vi "Create 2D Gauss.vi"(4 "Rauschen %":dbl=10.0, 6 "1/e HWidth":dbl, 7 "Y size":i32, 8 "mitte y":dbl, 9 "mitte x":dbl, 10 "Order":dbl, 11 "X size":i32) -> (1 "Total Count":sgl, 3 "2D Gauss":sgl[][](array[numeric]))   [LabVIEW 2020, in "Camera Simulator.lvlib"]
uses:
  Camera Simulator.lvlib
  <vilib>/numeric/Random Number (Range) DBL.vi
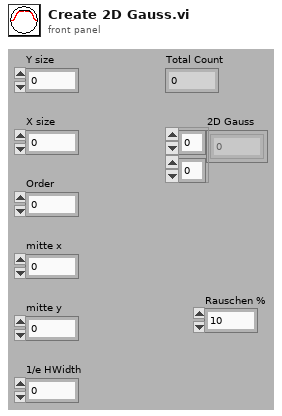
[diagram p1: front panel]
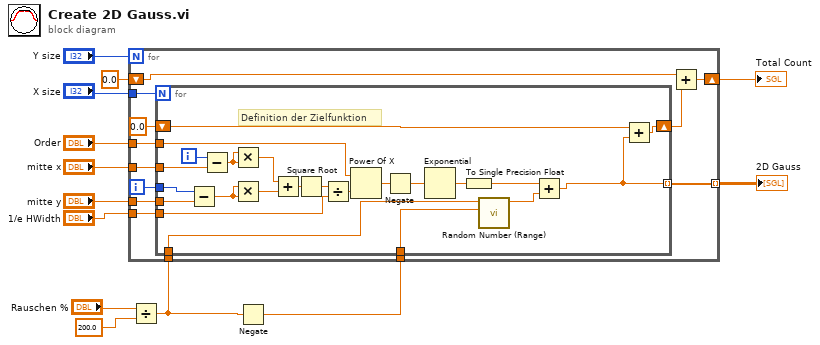
[diagram p0: block diagram]
diagram:
  n1 = Divide(x="Rauschen %", y=200.0) -> (x/y=w1:dbl)
  n2 = Negate(x=w1) -> (-x=w2:dbl)
  n3 = for {
    N: "Y size" -> [_]
    tunnel: "mitte x" -> [w26]
    tunnel: "mitte y" -> [w25]
    tunnel: "1/e HWidth" -> [w23]
    tunnel: "Order" -> [w22]
    tunnel: [w21] -> w6 mode=indexing
    tunnel: "X size" -> [w20]
    shift-right: [w18] -> w5
    shift-left: sgl 0.0 -> [w17]
    tunnel: w1 -> [w15]
    tunnel: w2 -> [w14]
    i -> [w24]
    n4 = for {
      N: w20 -> [_]
      tunnel: w26 -> [w48]
      tunnel: w25 -> [w46]
      tunnel: w24 -> [w47]
      tunnel: w23 -> [w45]
      tunnel: w22 -> [w43]
      tunnel: [w30] -> w21 mode=indexing
      shift-right: [w32] -> w19
      shift-left: sgl 0.0 -> [w31]
      tunnel: w15 -> [w29]
      tunnel: w14 -> [w28]
      i -> [w49]
      # "Definition der Zielfunktion"
      n5 = Subtract(x=w47, y=w46) -> (x-y=w39:dbl)
      n6 = Subtract(x=w49, y=w48) -> (x-y=w40:dbl)
      n7 = Multiply(x=w40, y=w40) -> (x*y=w37:dbl)
      n8 = Multiply(x=w39, y=w39) -> (x*y=w38:dbl)
      n9 = Add(x=w37, y=w38) -> (x+y=w36:dbl)
      n10 = Square Root(x=w36) -> (sqrt(x)=w35:dbl)
      n11 = Divide(x=w35, y=w45) -> (x/y=w44:dbl)
      n12 = Power Of X(1:w44, 2:w43) -> (0:w41:dbl)
      n13 = Negate(x=w41) -> (-x=w34:dbl)
      n14 = Exponential(1:w34) -> (0:w42:dbl)
      n15 = To Single Precision Float(number=w42) -> (single precision float=w33:sgl)
      n16 = call-poly <vilib>:"Random Number (Range).vi"("lower bound (0)"=w28, "upper bound (100)"=w29) -> ("number"=w27:dbl)  [unwired: 9 in]
      n17 = Add(x=w33, y=w27) -> (x+y=w30:dbl)
      n18 = Add(x=w31, y=w30) -> (x+y=w32:dbl)
    }
    n19 = Add(x=w17, y=w19) -> (x+y=w18:dbl)
  }
  "2D Gauss" <- w6
  "Total Count" <- w5
